vi "compare.vi"() -> ()   [LabVIEW 2020]
panel:
  in  "y":dbl
  in  "x":dbl
  out "x >= y?":bool
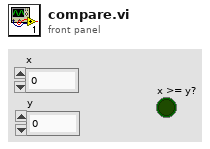
[diagram p1: front panel]
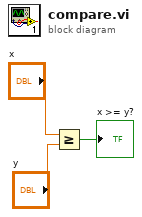
[diagram p0: block diagram]
diagram:
  n1 = Greater Or Equal?(x="x", y="y") -> (x >= y?=→"x >= y?":bool)
